vi "DIOChange.vi"(3 "Changed DIO Tydef":T1, 5 "Experiment State in":T2={"error"={"status"=FALSE, "code"=0, "source"=""}, "Digitizer DAQmx Tasks"={"TaskArray"=[]}, "DAQ Settings"={"Channel Settings"=[], "Card Settings"=[]}, "Synchronization Settings"={"Synchronizer 0"="", "source terminal"="", "Synchronizer 1"="PXI1Slot2"}, "DAQ Data"=[], "Next Shot#"="", "System Message"="", "User Shot Notes"="", "Timing Settings"={"Timing Card Settings"=[], "Timing Channel Settings"=[]}, "Timing Tasks"={"TaskArray"=[]}, "Tree"="", "Time Card/Channels"=[], "DAQ Card/Channels"=[], "Program Version"="", "RIO Settings"={"Channel Settings"=[], "Card Settings"=[]}, "RIO References"={"Reference Array"=[]}, "RIO Data"={"RIO Deleaved Data"=[], "Raw Readout"=[]}, "RIO Card/Channels"=[3, 8], "DIO Channels"=0, "DIO Settings"={"DIO Channel Array"=[]}, "Tachometer Controls"={"Tach Calibration folder"=path "Z:/Data/Calibration/Tachometer", "PSU2 charging Voltage [kV]"=0.0, "PSU2 Counter"="", "PSU2 task"="PSU2", "PSU3 Counter"="", "PSU3 task"="", "PSU3 charging Voltage [kV]"=0.0}, "Global Settings"={"Initial Background Values"={"Reference Shot #"=0.0, "Background pressure [Torr]"=0.0, "Cryo temp [V]"=0.0, "Cryo temp [K]"=0.0}, "Gas Puffing"={"Gas A type"="N", "Gas B type"="N", "Gas C type"="N", "Gas A pressure [psi]"=0.0, "Gas B pressure [psi]"=0.0, "Gas C pressure [psi]"=0.0, "Innner Electrode"="", "Middle Electrode"="", "Outer Electrode"="", "Gas A bottle pressure [psi]"=0.0, "Gas B bottle pressure [psi]"=0.0, "Gas C bottle pressure [psi]"=0.0}, "PSU Voltages"={"Bias1 Voltage [V]"=0.0, "Bias2 Voltage [V]"=0.0, "PSU1 Voltage [V]"=0.0, "Puff-PSU1 CH1 Voltage [V]"=0.0, "Puff-PSU1 CH2 Voltage [V]"=0.0, "Puff-PSU1 CH3 Voltage [V]"=0.0}, "Scope Details"={"CH1"="", "CH2"="", "CH3"="", "CH4"="", "CH1 Ground State"="Grounded", "CH2 Ground State"="Grounded", "CH3 Ground State"="Grounded", "CH4 Ground State"="Grounded"}}} {"RIO Settings"."Card Settings"."Sample Rate" format="%#_3p"; "Timing Settings"."Timing Channel Settings"."FrontPanelTime" format="%.3p"; "Timing Settings"."Timing Channel Settings"."Pulse width (s)" format="%.3p"; "Timing Settings"."Timing Channel Settings"."Delay (s)" format="%.3p"; "DAQ Settings"."Card Settings"."Global Edge Type" items=["Rising"=10280, "Falling"=10171]; "DAQ Settings"."Card Settings"."Sample Rate" format="%#_3p"}) -> (2 "Experiment State out":T2={"error"={"status"=FALSE, "code"=0, "source"=""}, "Digitizer DAQmx Tasks"={"TaskArray"=[]}, "DAQ Settings"={"Channel Settings"=[], "Card Settings"=[]}, "Synchronization Settings"={"Synchronizer 0"="", "source terminal"="", "Synchronizer 1"="PXI1Slot2"}, "DAQ Data"=[], "Next Shot#"="", "System Message"="", "User Shot Notes"="", "Timing Settings"={"Timing Card Settings"=[], "Timing Channel Settings"=[]}, "Timing Tasks"={"TaskArray"=[]}, "Tree"="", "Time Card/Channels"=[], "DAQ Card/Channels"=[], "Program Version"="", "RIO Settings"={"Channel Settings"=[], "Card Settings"=[]}, "RIO References"={"Reference Array"=[]}, "RIO Data"={"RIO Deleaved Data"=[], "Raw Readout"=[]}, "RIO Card/Channels"=[3, 8], "DIO Channels"=0, "DIO Settings"={"DIO Channel Array"=[]}, "Tachometer Controls"={"Tach Calibration folder"=path "Z:/Data/Calibration/Tachometer", "PSU2 charging Voltage [kV]"=0.0, "PSU2 Counter"="", "PSU2 task"="PSU2", "PSU3 Counter"="", "PSU3 task"="", "PSU3 charging Voltage [kV]"=0.0}, "Global Settings"={"Initial Background Values"={"Reference Shot #"=0.0, "Background pressure [Torr]"=0.0, "Cryo temp [V]"=0.0, "Cryo temp [K]"=0.0}, "Gas Puffing"={"Gas A type"="N", "Gas B type"="N", "Gas C type"="N", "Gas A pressure [psi]"=0.0, "Gas B pressure [psi]"=0.0, "Gas C pressure [psi]"=0.0, "Innner Electrode"="", "Middle Electrode"="", "Outer Electrode"="", "Gas A bottle pressure [psi]"=0.0, "Gas B bottle pressure [psi]"=0.0, "Gas C bottle pressure [psi]"=0.0}, "PSU Voltages"={"Bias1 Voltage [V]"=0.0, "Bias2 Voltage [V]"=0.0, "PSU1 Voltage [V]"=0.0, "Puff-PSU1 CH1 Voltage [V]"=0.0, "Puff-PSU1 CH2 Voltage [V]"=0.0, "Puff-PSU1 CH3 Voltage [V]"=0.0}, "Scope Details"={"CH1"="", "CH2"="", "CH3"="", "CH4"="", "CH1 Ground State"="Grounded", "CH2 Ground State"="Grounded", "CH3 Ground State"="Grounded", "CH4 Ground State"="Grounded"}}} {"RIO Settings"."Card Settings"."Sample Rate" format="%#_3p"; "Timing Settings"."Timing Channel Settings"."FrontPanelTime" format="%.3p"; "Timing Settings"."Timing Channel Settings"."Pulse width (s)" format="%.3p"; "Timing Settings"."Timing Channel Settings"."Delay (s)" format="%.3p"; "DAQ Settings"."Card Settings"."Global Edge Type" items=["Rising"=10280, "Falling"=10171]; "DAQ Settings"."Card Settings"."Sample Rate" format="%#_3p"})   [LabVIEW 2014]
doc: "Handle DIO changes identified in the producer."
uses:
  Controls/ExperimentStateCluster.ctl
  Controls/DigitizerSettingsChannelSettings.ctl
  Controls/DigitizerSettingsCardSettingsArray.ctl
  Controls/DigitizerSettingsCardSettings.ctl
  Controls/TimingSettings.ctl
  Controls/TimingCardSettings.ctl
  Controls/TimingChannelSettings.ctl
  Controls/RIOSettingsExperimentStateCluster.ctl
  Controls/RIOChannelSettingsArrayExperimentStateCluster.ctl
  Controls/RIOSettingsChannelSettings.ctl
  Controls/RIOSettingsCardSettingsArray.ctl
  Controls/RIOSettingsCardSettings.ctl
  <vilib>/userdefined/High Color/nirio_resource_hc.ctl
  Controls/RIOData.ctl
  Controls/DIOChannel.ctl
  Controls/TachometerControls.ctl
  Controls/Global Settings/GlobalSettings.ctl
  Controls/Global Settings/InitialBackgroundValues.ctl
  Controls/Global Settings/GasPuffing.ctl
  Controls/Global Settings/PSUVoltages.ctl
  Controls/Global Settings/ScopeDetails.ctl
  Controls/ChangedDIOTypdef.ctl
  <vilib>/DAQmx/create/channels.llb/DAQmx Create Channel (DO-Digital Output).vi
  <vilib>/DAQmx/write.llb/DAQmx Write (Digital Bool 1Line 1Point).vi
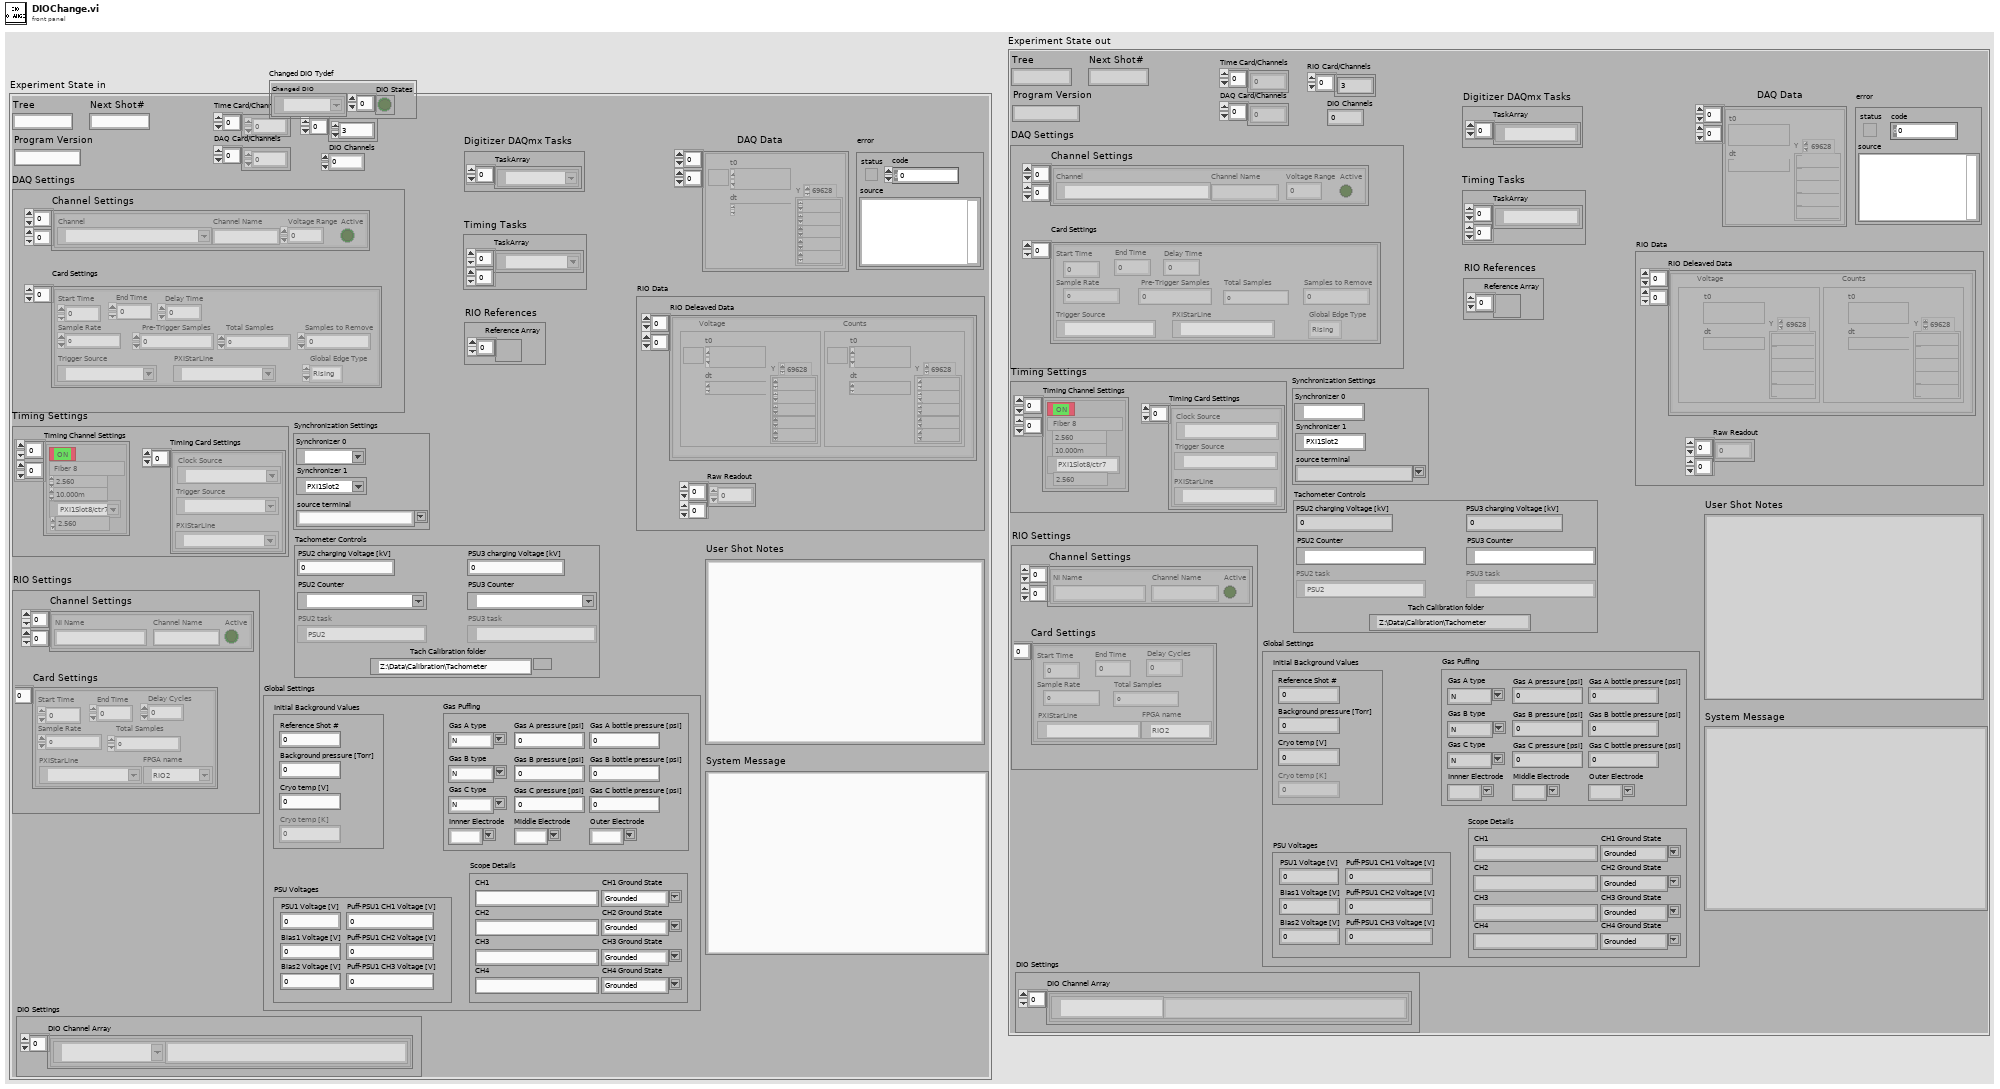
[diagram p1: front panel]
types:
  T1 = typedef "ChangedDIOTypdef.ctl" = cluster{"Changed DIO":tag[], "DIO States":bool[]}
  T2 = typedef "ExperimentStateCluster.ctl" = cluster{"error":errorcluster, "Digitizer DAQmx Tasks":cluster{"TaskArray":refnum<k21>[]}, "DAQ Settings":cluster{"Channel Settings":T3[][], "Card Settings":T4}, "Synchronization Settings":cluster{"Synchronizer 0":refnum<k15>, "source terminal":string, "Synchronizer 1":refnum<k15>}, "DAQ Data":waveform(dbl)[][], "Next Shot#":string, "System Message":string, "User Shot Notes":string, "Timing Settings":T6, "Timing Tasks":cluster{"TaskArray":refnum<k21>[][]}, "Tree":string, "Time Card/Channels":i32[], "DAQ Card/Channels":i32[], "Program Version":string, "RIO Settings":T9, "RIO References":cluster{"Reference Array":refnum<k20>[]}, "RIO Data":T15, "RIO Card/Channels":i32[], "DIO Channels":i32, "DIO Settings":cluster{"DIO Channel Array":T16[]}, "Tachometer Controls":T17, "Global Settings":T18}
  T3 = typedef "DigitizerSettingsChannelSettings.ctl" = cluster{"Channel":tag, "Channel Name":string, "Voltage Range":dbl, "Active":bool}
  T4 = typedef "DigitizerSettingsCardSettingsArray.ctl" = T5[]
  T5 = typedef "DigitizerSettingsCardSettings.ctl" = cluster{"Start Time":dbl, "End Time":dbl, "Sample Rate":dbl, " Pre-Trigger Samples":u32, "Total Samples":i32, "Samples to Remove":u32, "Trigger Source":tag, "Global Edge Type":i32, "PXIStarLine":tag, "Delay Time":dbl}
  T6 = typedef "TimingSettings.ctl" = cluster{"Timing Card Settings":T7[], "Timing Channel Settings":T8[][]}
  T7 = typedef "TimingCardSettings.ctl" = cluster{"Trigger Source":tag, "Clock Source":tag, "PXIStarLine":tag}
  T8 = typedef "TimingChannelSettings.ctl" = cluster{"Delay (s)":dbl, "Pulse width (s)":dbl, "Active":bool, "Channel Name":string, "counter":tag, "FrontPanelTime":dbl}
  T9 = typedef "RIOSettingsExperimentStateCluster.ctl" = cluster{"Channel Settings":T10, "Card Settings":T12}
  T10 = typedef "RIOChannelSettingsArrayExperimentStateCluster.ctl" = T11[][]
  T11 = typedef "RIOSettingsChannelSettings.ctl" = cluster{"Channel Name":string, "Active":bool, "NI Name":string}
  T12 = typedef "RIOSettingsCardSettingsArray.ctl" = T13[]
  T13 = typedef "RIOSettingsCardSettings.ctl" = cluster{"Start Time":dbl, "End Time":dbl, "Sample Rate":dbl, "Total Samples":u64, "PXIStarLine":tag, "Delay Cycles":u64, "FPGA name":T14}
  T14 = typedef "nirio_resource_hc.ctl" = tag
  T15 = typedef "RIOData.ctl" = cluster{"RIO Deleaved Data":cluster{"Voltage":waveform(dbl), "Counts":waveform(i16)}[][], "Raw Readout":u64[][]}
  T16 = typedef "DIOChannel.ctl" = cluster{"Channel Name":string, "NI Name":tag}
  T17 = typedef "TachometerControls.ctl" = cluster{"Tach Calibration folder":path, "PSU2 charging Voltage [kV]":dbl, "PSU2 Counter":tag, "PSU2 task":refnum<k21>, "PSU3 Counter":tag, "PSU3 task":refnum<k21>, "PSU3 charging Voltage [kV]":dbl}
  T18 = typedef "GlobalSettings.ctl" = cluster{"Initial Background Values":T19, "Gas Puffing":T20, "PSU Voltages":T21, "Scope Details":T22}
  T19 = typedef "InitialBackgroundValues.ctl" = cluster{"Reference Shot #":dbl, "Background pressure [Torr]":dbl, "Cryo temp [V]":dbl, "Cryo temp [K]":dbl}
  T20 = typedef "GasPuffing.ctl" = cluster{"Gas A type":string, "Gas B type":string, "Gas C type":string, "Gas A pressure [psi]":dbl, "Gas B pressure [psi]":dbl, "Gas C pressure [psi]":dbl, "Innner Electrode":string, "Middle Electrode":string, "Outer Electrode":string, "Gas A bottle pressure [psi]":dbl, "Gas B bottle pressure [psi]":dbl, "Gas C bottle pressure [psi]":dbl}
  T21 = typedef "PSUVoltages.ctl" = cluster{"Bias1 Voltage [V]":dbl, "Bias2 Voltage [V]":dbl, "PSU1 Voltage [V]":dbl, "Puff-PSU1 CH1 Voltage [V]":dbl, "Puff-PSU1 CH2 Voltage [V]":dbl, "Puff-PSU1 CH3 Voltage [V]":dbl}
  T22 = typedef "ScopeDetails.ctl" = cluster{"CH1":string, "CH2":string, "CH3":string, "CH4":string, "CH1 Ground State":string, "CH2 Ground State":string, "CH3 Ground State":string, "CH4 Ground State":string}
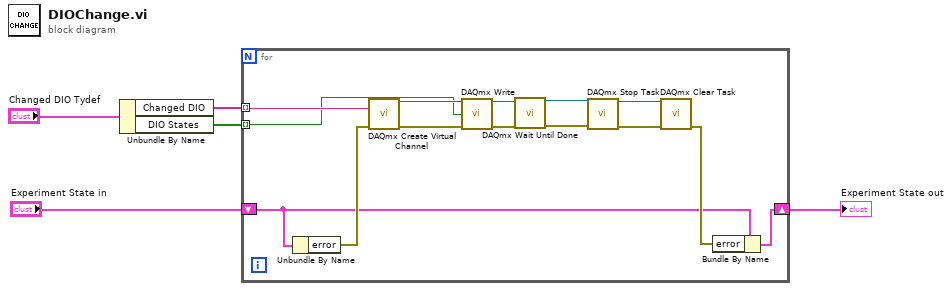
[diagram p0: block diagram]
diagram:
  n1 = Unbundle By Name("Changed DIO Tydef") -> ("Changed DIO"=w4:tag[], "DIO States"=w3:bool[])
  n2 = for {
    tunnel: w4 -> [w15] mode=indexing
    tunnel: w3 -> [w13] mode=indexing
    shift-right: [w7] -> w1
    shift-left: "Experiment State in" -> [w6]
    n3 = Unbundle By Name(w6) -> ("error"=w9:errorcluster)
    n4 = call-poly <vilib>:"DAQmx Create Virtual Channel.vi"("lines"=w15, "error in"=w9) -> ("task out"=w14:refnum<k21>, "error out"=w19:errorcluster)  [unwired: 12 in]
    n5 = call-poly <vilib>:"DAQmx Write.vi"("task/channels in"=w14, "data"=w13, "error in"=w19) -> ("task out"=w12:refnum<k21>, "error out"=w18:errorcluster)  [unwired: 1 in, 10 out]
    n6 = call <vilib>:"DAQmx Wait Until Done.vi"("task/channels in"=w12, "error in"=w18) -> ("task out"=w11:refnum<k21>, "error out"=w17:errorcluster)  [unwired: 12 in]
    n7 = call <vilib>:"DAQmx Stop Task.vi"("task/channels in"=w11, "error in"=w17) -> ("task out"=w10:refnum<k21>, "error out"=w16:errorcluster)  [unwired: 12 in]
    n8 = call <vilib>:"DAQmx Clear Task.vi"("task in"=w10, "error in"=w16) -> ("error out"=w8:errorcluster)  [unwired: 13 in]
    n9 = Bundle By Name(cluster=w6, "error"=w8) -> (w7:T2)
  }
  "Experiment State out" <- w1
